vi "sync_costas_loop.vi"(6 "arity":enum16{"binary", "quadrature"}(ring), 8 "loop bandwidth":dbl=0.0314 format="%#_13g", 11 "symbols":cdb[](array[numeric])) -> (3 "outputs":cdb[](array[numeric]))   [LabVIEW 2014]
uses:
  <vilib>/imath/engines/lvmath2/RunTimeEngine/NodeEndStatement/NIMS_NodeEndStatement_Output.vi
  <instcachedir>/0/NIMS_NodeEndStatement_Output_53EC0D466D134D7ABD903AC30B43404B.lvgen/NIMS_NodeEndStatement_Output_53EC0D466D134D7ABD903AC30B43404B_001.vi
  <vilib>/imath/engines/lvmath2/RunTimeEngine/ErrorHandling/NIMS_Finalize Error.vi
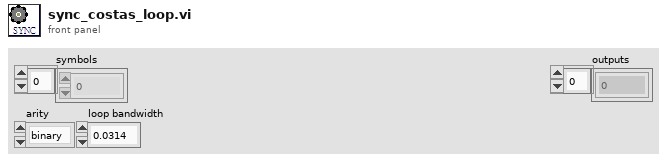
[diagram p1: front panel]
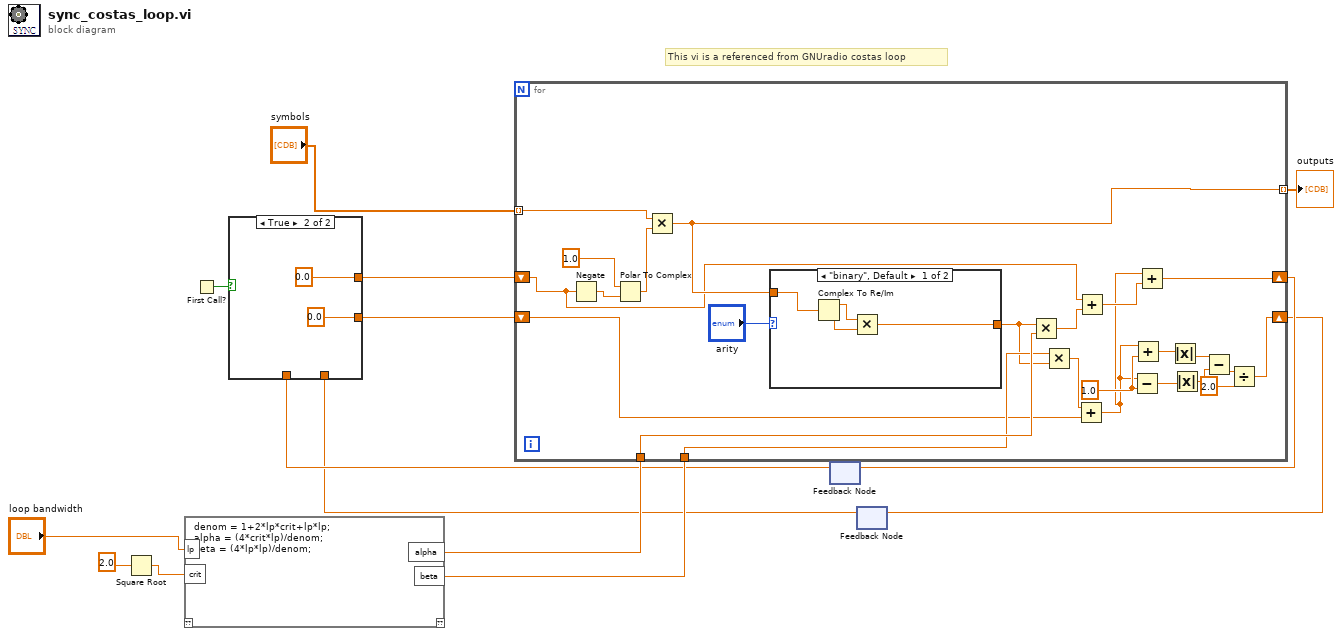
[diagram p0: block diagram]
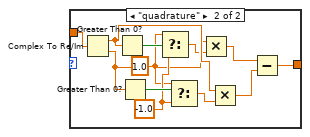
[diagram p3: hidden frame]
diagram:
  # "This vi is a referenced from GNUradio costas loop"
  n1 = Square Root(x=2.0) -> (sqrt(x)=w10:dbl)
  n2 = mathscript code="denom = 1+2*lp*crit+lp*lp;\nalpha = (4*crit*lp)/denom;\nbeta = (4*lp*lp)/denom;"("lp"="loop bandwidth", "crit"=w10) -> ("alpha"=w8:dbl, "beta"=w7:dbl)  [unwired: 1 in, 1 out]
  n3 = First Call?() -> (First Call?: T/F=w14:bool)
  n4 = feedback #1() -> (w3:dbl)  [unwired: 1 in]
  n5 = feedback #2() -> (w1:dbl)  [unwired: 1 in]
  n6 = case shown="True" w14 {
    tunnel: [w15 0.0] -> w13
    tunnel: [w16 0.0] -> w12
    tunnel: w3 -> [w15 _]
    tunnel: w1 -> [w16 _]
    frame False {
    }
    frame True {
    }
  }
  n7 = for {
    shift-right: [w19] -> w4
    shift-left: w13 -> [w24]
    shift-right: [w26] -> w2
    shift-left: w12 -> [w21]
    tunnel: w8 -> [w36]
    tunnel: w7 -> [w35]
    tunnel: "symbols" -> [w39] mode=indexing
    tunnel: [w37] -> w5 mode=indexing
    w31 = 1.0
    n8 = Negate(x=w24) -> (-x=w41:dbl)
    n9 = Polar To Complex(1:w41, 2:1.0) -> (0:w40:cdb)
    n10 = Multiply(x=w39, y=w40) -> (x*y=w37:cdb)
    n11 = case shown="\"binary\", Default" "arity" {
      tunnel: w37 -> [w46 w58]
      tunnel: [w43 w47] -> w34
      frame "binary", Default {
        n12 = Complex To Re/Im(x + iy=w46) -> (x=w45:dbl, y=w44:dbl)
        n13 = Multiply(x=w45, y=w44) -> (x*y=w43:dbl)
      }
      frame "quadrature" {
        w55 = -1.0
        w54 = 1.0
        n14 = Complex To Re/Im(x + iy=w58) -> (x=w52:dbl, y=w51:dbl)
        n15 = Greater Than 0?(x=w52) -> (x > 0?=w57:bool)
        n16 = Greater Than 0?(x=w51) -> (x > 0?=w56:bool)
        n17 = Select(t=w54, s=w57, f=w55) -> (s? t:f=w50:dbl)
        n18 = Select(t=w54, s=w56, f=w55) -> (s? t:f=w53:dbl)
        n19 = Multiply(x=w51, y=w50) -> (x*y=w49:dbl)
        n20 = Multiply(x=w52, y=w53) -> (x*y=w48:dbl)
        n21 = Subtract(x=w49, y=w48) -> (x-y=w47:dbl)
      }
    }
    n22 = Multiply(x=w34, y=w36) -> (x*y=w25:dbl)
    n23 = Multiply(x=w35, y=w34) -> (x*y=w22:dbl)
    n24 = Add(x=w22, y=w21) -> (x+y=w20:dbl)
    n25 = Add(x=w24, y=w25) -> (x+y=w23:dbl)
    n26 = Subtract(x=w20, y=w31) -> (x-y=w32:dbl)
    n27 = Add(x=w20, y=w31) -> (x+y=w33:dbl)
    n28 = Add(x=w20, y=w23) -> (x+y=w19:dbl)
    n29 = Absolute Value(x=w33) -> (abs(x)=w30:dbl)
    n30 = Absolute Value(x=w32) -> (abs(x)=w29:dbl)
    n31 = Subtract(x=w30, y=w29) -> (x-y=w28:dbl)
    n32 = Divide(x=w28, y=2.0) -> (x/y=w26:dbl)
  }
  "outputs" <- w5
  n33 = feedback-in #1(w4) -> ()
  n34 = feedback-in #2(w2) -> ()
